vi "PID Drive.vi"(0 "RobotDriveDevRef":T1={"DevStatus"={"status"=FALSE, "code"=0, "source"=""}, "Motors[]"=[], "Square Inputs"=FALSE, "Max Output"=1.0}, 1 "Distance (in)":dbl format="%.2f", 2 "Rotation (deg)":dbl, 3 "Wheel diameter (in)":dbl=6.0, 4 "Wheel Axel Width (in)":dbl, 6 "Right encoder renum":string="My Encoder RefNum", 8 "Left encoder refnum":string="My Encoder RefNum") -> ()   [LabVIEW 2014, in "hhVI.lvlib"]
doc: "Drives the robot based on a set distance or rotation."
uses:
  hhVI.lvlib
  <vilib>/Rock Robotics/WPI/RobotDrive/WPI_RobotDriveDevRef.ctl
  <vilib>/Rock Robotics/WPI/MotorControl/WPI_MotorControlDeviceRef.ctl
  <vilib>/Rock Robotics/WPI/MotorControl/WPI_MotorControlType.ctl
  <vilib>/Rock Robotics/SystemInterfaces/Typedef/FPGA_TypedefDigitalModule.ctl
  <vilib>/Rock Robotics/SystemInterfaces/DIO/FPGA_DIOPWMChannel.ctl
  <vilib>/Rock Robotics/WPI/PWM/WPI_PWMDeadband.ctl
  <vilib>/Rock Robotics/WPI/CAN/Jaguar/SubVIs/WPI_CANJaguar_ControlMode.ctl
  <vilib>/Rock Robotics/WPI/CAN/TalonSRX/WPI_CANTalonSRX_APIControlMode.ctl
  <vilib>/Rock Robotics/WPI/PWM/WPI_PWMTransform_ConPane.ctl
  <vilib>/addons/control/pid/pid.llb/PID (DBL).vi
  <vilib>/addons/control/pid/NI_PID_pid.lvlib
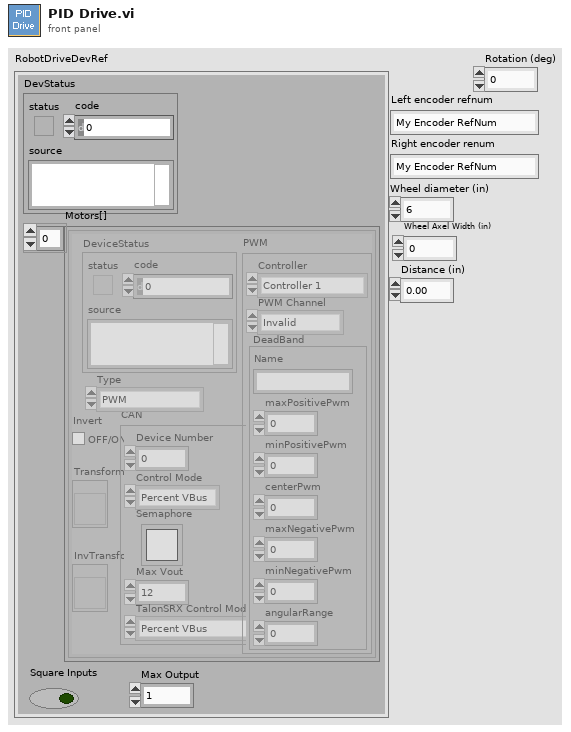
[diagram p1: front panel]
types:
  T1 = typedef "WPI_RobotDriveDevRef.ctl" = cluster{"DevStatus":errorcluster, "Motors[]":T2[], "Square Inputs":bool, "Max Output":dbl}
  T2 = typedef "WPI_MotorControlDeviceRef.ctl" = cluster{"DeviceStatus":errorcluster, "Type":T3, "PWM":cluster{"Controller":T4, "PWM Channel":T5, "DeadBand":T6}, "CAN":cluster{"Device Number":u8, "Control Mode":T7, "Semaphore":T8, "Max Vout":dbl, "TalonSRX Control Mode":T9}, "Invert":bool, "TransformRef":T10, "InvTransformRef":T10}
  T3 = typedef "WPI_MotorControlType.ctl" = enum16{"PWM", "CAN", "CANTalonSRX"}
  T4 = typedef "FPGA_TypedefDigitalModule.ctl" = enum16{"Controller 1"}
  T5 = typedef "FPGA_DIOPWMChannel.ctl" = enum8{"PWM 0", "PWM 1", "PWM 2", "PWM 3", "PWM 4", "PWM 5", "PWM 6", "PWM 7", "PWM 8", "PWM 9", "PWM MXP 0", "PWM MXP 1", "PWM MXP 2", "PWM MXP 3", "PWM MXP 4", "PWM MXP 5", "PWM MXP 6", "PWM MXP 7", "PWM MXP 8", "PWM MXP 9", "Invalid"}
  T6 = typedef "WPI_PWMDeadband.ctl" = cluster{"Name":string, "maxPositivePwm":i32, "minPositivePwm":i32, "centerPwm":i32, "maxNegativePwm":i32, "minNegativePwm":i32, "angularRange":u16}
  T7 = typedef "WPI_CANJaguar_ControlMode.ctl" = enum8{"Percent VBus", "Current", "Speed", "Position", "Voltage"}
  T8 = typedef "Semaphore RefNum" = refnum<k1>
  T9 = typedef "WPI_CANTalonSRX_APIControlMode.ctl" = enum8{"Percent VBus", "Speed", "Position", "Slave", "Unchanged / Invalid"}
  T10 = typedef "WPI_PWMTransform_ConPane.ctl" = refnum<vi>
  T11 = cluster{"proportional gain (Kc)":dbl, "integral time (Ti, min)":dbl, "derivative time (Td, min)":dbl}
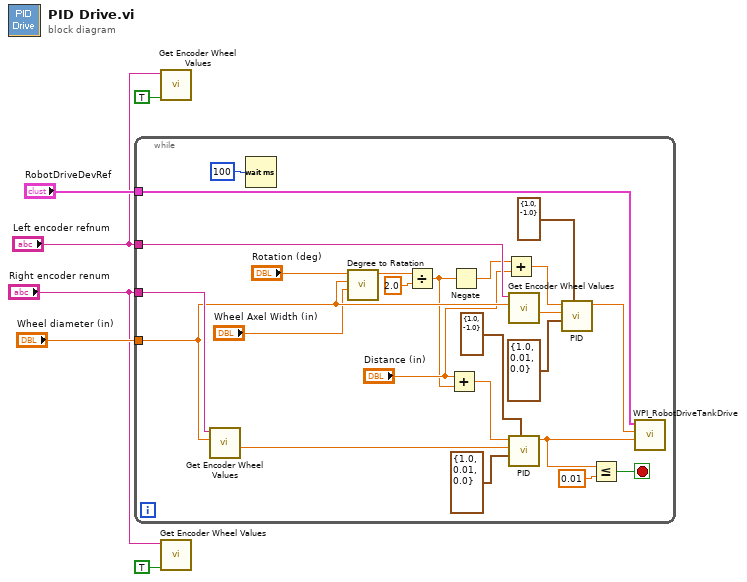
[diagram p0: block diagram]
diagram:
  n1 = while {
    tunnel: "RobotDriveDevRef" -> [w27]
    tunnel: "Left encoder refnum" -> [w22]
    tunnel: "Right encoder renum" -> [w21]
    tunnel: "Wheel diameter (in)" -> [w15]
    stop <- w19 stop-if-true
    n2 = call "Get Encoder Wheel Values.vi"("Wheel diameter (in)"=w15, "refnum name"=w21) -> ("Distance (in)"=w23:dbl)  [unwired: 4 in, 5 out]
    n3 = Wait (ms)(milliseconds to wait=u32 100) -> ()  [unwired: 1 out]
    n4 = call "Degree to Ratation.vi"("Wheel Axel Width (in)"="Wheel Axel Width (in)", "Wheel Diameter (in)"=w15, "Rotation (degrees)"="Rotation (deg)") -> ("Rotations needed"=w13:dbl)  [unwired: 8 in]
    n5 = Divide(x=w13, y=2.0) -> (x/y=w9:dbl)
    n6 = Add(x="Distance (in)", y=w9) -> (x+y=w7:dbl)
    n7 = Negate(x=w9) -> (-x=w11:dbl)
    n8 = Add(x=w11, y="Distance (in)") -> (x+y=w8:dbl)
    n9 = call "Get Encoder Wheel Values.vi"("Wheel diameter (in)"=w15, "refnum name"=w22) -> ("Distance (in)"=w29:dbl)  [unwired: 4 in, 5 out]
    n10 = call-poly <vilib>:"PID.vi"("output range"=cluster{"output high":dbl, "output low":dbl} {"output high"=1.0, "output low"=-1.0}, "PID gains"=T11 {"proportional gain (Kc)"=1.0, "integral time (Ti, min)"=0.01, "derivative time (Td, min)"=0.0}, "process variable"=w23, "setpoint"=w7) -> ("output"=w18:dbl)  [unwired: 6 in, 1 out]
    n11 = call-poly <vilib>:"PID.vi"("output range"=cluster{"output high":dbl, "output low":dbl} {"output high"=1.0, "output low"=-1.0}, "PID gains"=T11 {"proportional gain (Kc)"=1.0, "integral time (Ti, min)"=0.01, "derivative time (Td, min)"=0.0}, "process variable"=w29, "setpoint"=w8) -> ("output"=w28:dbl)  [unwired: 6 in, 1 out]
    n12 = Less Or Equal?(x=w18, y=0.01) -> (x <= y?=w19:bool)
    n13 = call <vilib>:"WPI_RobotDriveTankDrive.vi"("Right axis value"=w18, "Left axis value"=w28, "RobotDriveDevRef"=w27) -> ()  [unwired: 6 in, 3 out]
  }
  n14 = call "Get Encoder Wheel Values.vi"("Reset encoder"=TRUE ("Reset Encoder"), "refnum name"="Left encoder refnum") -> ()  [unwired: 4 in, 6 out]
  n15 = call "Get Encoder Wheel Values.vi"("Reset encoder"=TRUE ("Reset Encoder"), "refnum name"="Right encoder renum") -> ()  [unwired: 4 in, 6 out]
